vi "Pointer producer consumer help.vi"() -> ()   [LabVIEW 2014]
panel:
  in  "Stop help":bool
  in  "Help Item":u16(ring) items=["Control Help", "Display Help", "Graph Help"]
  out "Help Image":picture
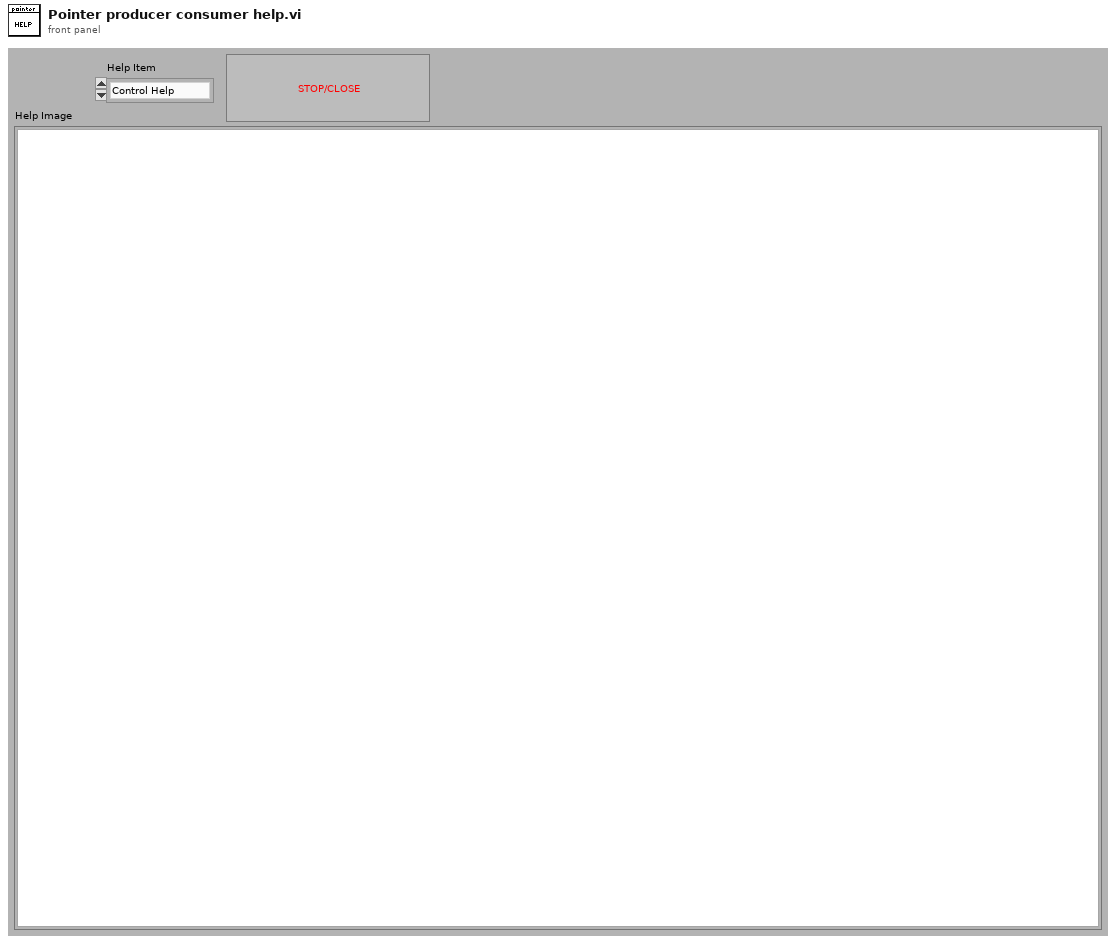
[diagram p1: front panel]
types:
  T1 = typedef "imagedata.ctl" = cluster{"image type":i32, "image depth":i32, "image":u8[], "mask":u8[], "colors":u32[], "Rectangle":cluster{"left":i16, "top":i16, "right":i16, "bottom":i16}}
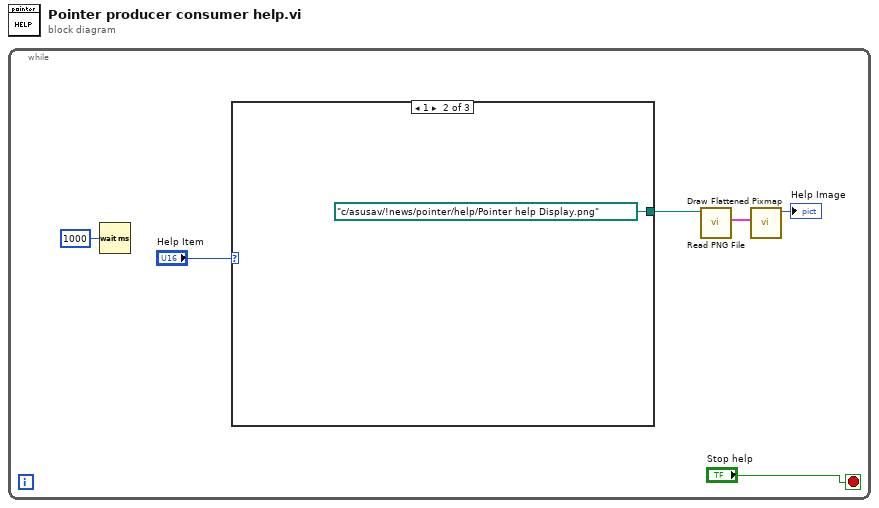
[diagram p0: block diagram]
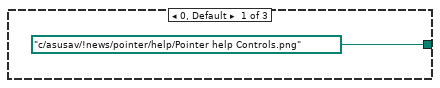
[diagram p2: hidden frame]
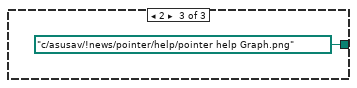
[diagram p3: hidden frame]
diagram:
  n1 = while {
    stop <- "Stop help" stop-if-true
    n2 = Wait (ms)(milliseconds to wait=u32 1000) -> ()  [unwired: 1 out]
    n3 = case shown="1" "Help Item" {
      tunnel: [path "c:/asusav/!news/pointer/help/Pointer help Controls.png" ("path to JPEG file") path "c:/asusav/!news/pointer/help/Pointer help Display.png" ("path to JPEG file") path "c:/asusav/!news/pointer/help/pointer help Graph.png" ("path to JPEG file")] -> w4
      frame 0, Default {
      }
      frame 1 {
      }
      frame 2 {
      }
    }
    n4 = call <vilib>:"Read PNG File.vi"("path to PNG file"=w4) -> ("image data"=w3:T1)  [unwired: 8 in, 2 out]
    n5 = call <vilib>:"Draw Flattened Pixmap.vi"("image data"=w3) -> ("new picture"=→"Help Image":picture)  [unwired: 8 in]
  }
